vi "Classical WSA (SubVI).vi"(7 "Select Method":T2(ring), 9 "Zc (mmHg/ml/s)":dbl, 10 "Flow Rate (ml/s)":waveform(dbl), 11 "Pressure (mmHg)":waveform(dbl)) -> (3 "WSA Waveforms":T1)   [LabVIEW 2017]
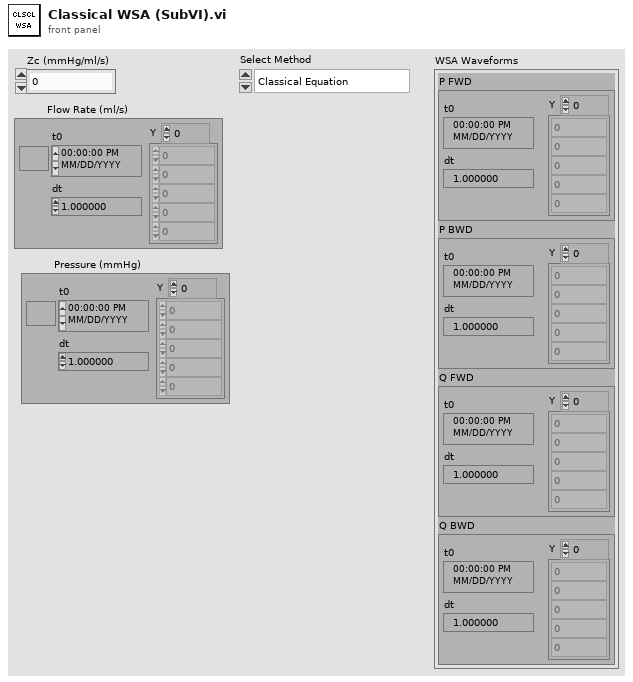
[diagram p1: front panel]
types:
  T1 = cluster{"P FWD":waveform(dbl), "P BWD":waveform(dbl), "Q FWD":waveform(dbl), "Q BWD":waveform(dbl)}
  T2 = enum16{"Classical Equation", "Succusive Wavefronts"}
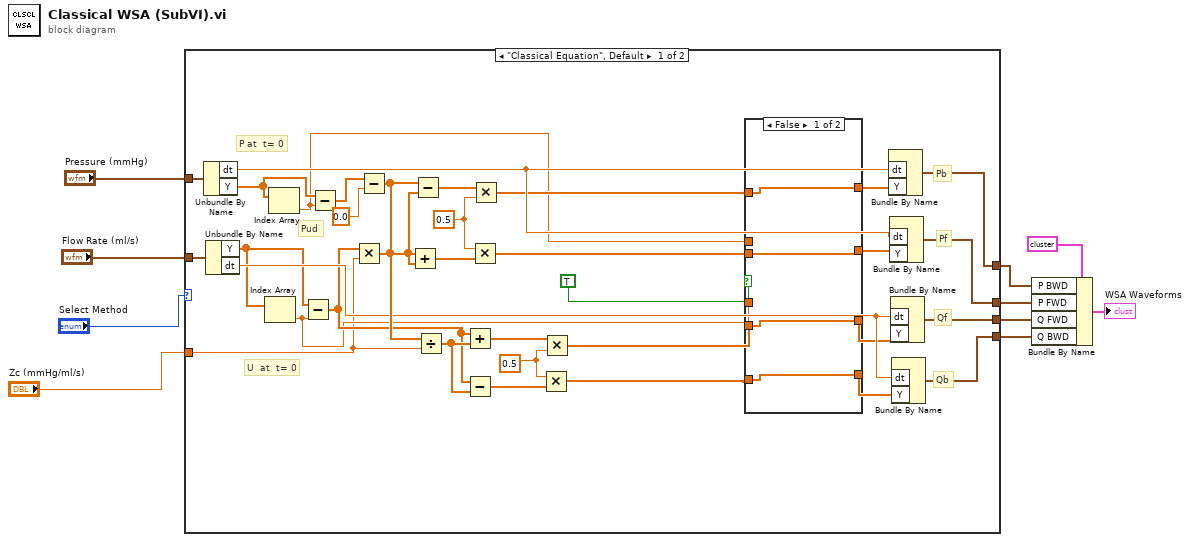
[diagram p0: block diagram]
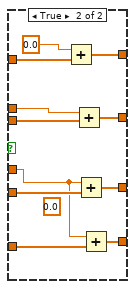
[diagram p2: hidden frame]
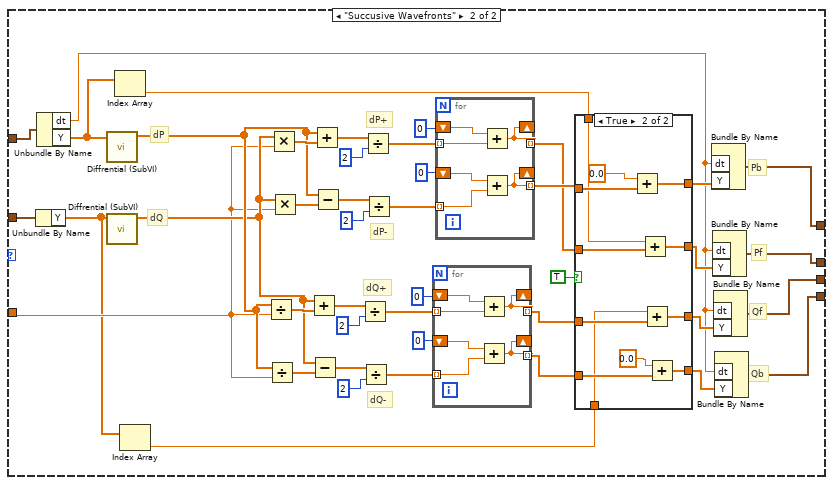
[diagram p3: hidden frame]
diagram:
  n1 = case shown="\"Classical Equation\", Default" "Select Method" {
    tunnel: [w44 w102] -> w9
    tunnel: [w43 w101] -> w8
    tunnel: [w42 w100] -> w7
    tunnel: [w41 w99] -> w6
    tunnel: "Pressure (mmHg)" -> [w13 w97]
    tunnel: "Flow Rate (ml/s)" -> [w12 w98]
    tunnel: "Zc (mmHg/ml/s)" -> [w11 w74]
    frame "Classical Equation", Default {
      w34 = 0.5 ("y")
      w32 = 0.5 ("y")
      # "U  at  t= 0"
      # "Pud"
      # "P at  t= 0"
      # "Qb"
      # "Qf"
      # "Pf"
      # "Pb"
      n2 = Unbundle By Name(w13) -> ("dt"=w38:dbl, "Y"=w29:dbl[])
      n3 = Unbundle By Name(w12) -> ("Y"=w27:dbl[], "dt"=w30:dbl)
      n4 = Index Array(array=w27) -> (element=w15:dbl)  [unwired: 1 in]
      n5 = Index Array(array=w29) -> (element=w21:dbl)  [unwired: 1 in]
      n6 = Subtract(x=w27, y=w15) -> (x-y=w26:dbl[])
      n7 = Subtract(x=w29, y=w21) -> (x-y=w28:dbl[])
      n8 = Multiply(x=w26, y=w11) -> (x*y=w40:dbl[])
      n9 = Subtract(x=w28, y=0.0) -> (x-y=w37:dbl[])
      n10 = Add(x=w37, y=w40) -> (x+y=w31:dbl[])
      n11 = Subtract(x=w37, y=w40) -> (x-y=w39:dbl[])
      n12 = Divide(x=w37, y=w11) -> (x/y=w36:dbl[])
      n13 = Add(x=w26, y=w36) -> (x+y=w35:dbl[])
      n14 = Subtract(x=w26, y=w36) -> (x-y=w33:dbl[])
      n15 = Multiply(x=w32, y=w31) -> (x*y=w22:dbl[])
      n16 = Multiply(x=w39, y=w32) -> (x*y=w24:dbl[])
      n17 = Multiply(x=w34, y=w33) -> (x*y=w17:dbl[])
      n18 = Multiply(x=w35, y=w34) -> (x*y=w19:dbl[])
      n19 = case shown="False" TRUE {
        tunnel: w24 -> [w48 w59]
        tunnel: [w48 w58] -> w23
        tunnel: w22 -> [w47 w56]
        tunnel: w21 -> [_ w55]
        tunnel: [w47 w54] -> w20
        tunnel: w19 -> [w46 w53]
        tunnel: [w46 w52] -> w18
        tunnel: w17 -> [w45 w51]
        tunnel: [w45 w50] -> w16
        tunnel: w15 -> [_ w49]
        frame False {
        }
        frame True {
          (unwired) 0.0
          n20 = Add(x=0.0, y=w59) -> (x+y=w58:dbl[])
          n21 = Add(x=w55, y=w56) -> (x+y=w54:dbl[])
          n22 = Add(x=w49, y=w53) -> (x+y=w52:dbl[])
          n23 = Add(x=w49, y=w51) -> (x+y=w50:dbl[])
        }
      }
      n24 = Bundle By Name("dt"=w38, "Y"=w23) -> (w44:waveform(dbl))  [unwired: 1 in]
      n25 = Bundle By Name("dt"=w38, "Y"=w20) -> (w43:waveform(dbl))  [unwired: 1 in]
      n26 = Bundle By Name("dt"=w30, "Y"=w18) -> (w42:waveform(dbl))  [unwired: 1 in]
      n27 = Bundle By Name("dt"=w30, "Y"=w16) -> (w41:waveform(dbl))  [unwired: 1 in]
    }
    frame "Succusive Wavefronts" {
      # "dQ"
      # "dP"
      # "dQ-"
      # "dQ+"
      # "dP-"
      # "dP+"
      # "Qb"
      # "Qf"
      # "Pf"
      # "Pb"
      n28 = Unbundle By Name(w98) -> ("Y"=w68:dbl[])
      n29 = Unbundle By Name(w97) -> ("dt"=w60:dbl, "Y"=w72:dbl[])
      n30 = call "Diffrential (SubVI).vi"("d(n)"=w72) -> ("d(n)-d(n+1)"=w76:dbl[])  [unwired: 10 in]
      n31 = call "Diffrential (SubVI).vi"("d(n)"=w68) -> ("d(n)-d(n+1)"=w75:dbl[])  [unwired: 10 in]
      n32 = Index Array(array=w72) -> (element=w71:dbl)  [unwired: 1 in]
      n33 = Index Array(array=w68) -> (element=w67:dbl)  [unwired: 1 in]
      n34 = Divide(x=w76, y=w74) -> (x/y=w86:dbl[])
      n35 = Divide(x=w76, y=w74) -> (x/y=w81:dbl[])
      n36 = Multiply(x=w75, y=w74) -> (x*y=w87:dbl[])
      n37 = Multiply(x=w75, y=w74) -> (x*y=w92:dbl[])
      n38 = Add(x=w75, y=w86) -> (x+y=w85:dbl[])
      n39 = Subtract(x=w75, y=w81) -> (x-y=w82:dbl[])
      n40 = Add(x=w76, y=w87) -> (x+y=w88:dbl[])
      n41 = Subtract(x=w76, y=w92) -> (x-y=w91:dbl[])
      n42 = Divide(x=w85, y=2 ("x")) -> (x/y=w80:dbl[])
      n43 = Divide(x=w82, y=2 ("x")) -> (x/y=w79:dbl[])
      n44 = Divide(x=w88, y=2 ("x")) -> (x/y=w93:dbl[])
      n45 = Divide(x=w91, y=2 ("x")) -> (x/y=w94:dbl[])
      n46 = for {
        tunnel: w80 -> [w124] mode=indexing
        tunnel: w79 -> [w121] mode=indexing
        shift-right: [w122] -> _
        shift-left: 0 ("x") -> [w123]
        tunnel: [w122] -> w66 mode=indexing
        shift-right: [w120] -> _
        shift-left: 0 ("x") -> [w119]
        tunnel: [w120] -> w65 mode=indexing
        n47 = Add(x=w123, y=w124) -> (x+y=w122:dbl)
        n48 = Add(x=w119, y=w121) -> (x+y=w120:dbl)
      }
      n49 = for {
        tunnel: w93 -> [w130] mode=indexing
        tunnel: w94 -> [w127] mode=indexing
        shift-right: [w128] -> _
        shift-left: 0 ("x") -> [w129]
        tunnel: [w128] -> w69 mode=indexing
        shift-right: [w126] -> _
        shift-left: 0 ("x") -> [w125]
        tunnel: [w126] -> w70 mode=indexing
        n50 = Add(x=w129, y=w130) -> (x+y=w128:dbl)
        n51 = Add(x=w125, y=w127) -> (x+y=w126:dbl)
      }
      n52 = case shown="True" TRUE {
        tunnel: w70 -> [w106 w118]
        tunnel: [w106 w117] -> w64
        tunnel: w69 -> [w105 w115]
        tunnel: [w105 w114] -> w63
        tunnel: w66 -> [w104 w113]
        tunnel: [w104 w112] -> w62
        tunnel: w65 -> [w103 w111]
        tunnel: [w103 w110] -> w61
        tunnel: w71 -> [_ w109]
        tunnel: w67 -> [_ w107]
        frame False {
        }
        frame True {
          n53 = Add(x=0.0, y=w118) -> (x+y=w117:dbl[])
          n54 = Add(x=w109, y=w115) -> (x+y=w114:dbl[])
          n55 = Add(x=w107, y=w113) -> (x+y=w112:dbl[])
          n56 = Add(x=0.0, y=w111) -> (x+y=w110:dbl[])
        }
      }
      n57 = Bundle By Name("dt"=w60, "Y"=w64) -> (w102:waveform(dbl))  [unwired: 1 in]
      n58 = Bundle By Name("dt"=w60, "Y"=w63) -> (w101:waveform(dbl))  [unwired: 1 in]
      n59 = Bundle By Name("dt"=w60, "Y"=w62) -> (w100:waveform(dbl))  [unwired: 1 in]
      n60 = Bundle By Name("dt"=w60, "Y"=w61) -> (w99:waveform(dbl))  [unwired: 1 in]
    }
  }
  n61 = Bundle By Name(cluster=T1 {"P FWD"={"t0"=timestamp(0 s since 1904-01-01), "dt"=1.0, "Y"=[]}, "P BWD"={"t0"=timestamp(0 s since 1904-01-01), "dt"=1.0, "Y"=[]}, "Q FWD"={"t0"=timestamp(0 s since 1904-01-01), "dt"=1.0, "Y"=[]}, "Q BWD"={"t0"=timestamp(0 s since 1904-01-01), "dt"=1.0, "Y"=[]}} ("Output Waveforms"), "P BWD"=w9, "P FWD"=w8, "Q FWD"=w7, "Q BWD"=w6) -> (→"WSA Waveforms":T1)
